vi "SW_Load_parameter_group_3.vi"(0 "Settings file refnum in":T2, 5 "Researcher name in":string, 7 "Settings parameter name":T1, 11 "error in":errorcluster) -> (4 "Settings file refnum out":T2, 6 "Researcher name out":string, 8 "Found?":bool, 10 "Group (section) cluster data out":variant, 15 "error out":errorcluster)   [LabVIEW 2018, in "Tracker.lvlib"]
uses:
  Tracker.lvlib
  <vilib>/Utility/config.llb/Config Data RefNum.ctl
  Controls/CTL_Settings_parameter_group_enum.ctl
  Controls/CTL_Settings_cluster.ctl
  Controls/CTL_Histogram_parameters.ctl
  Controls/CTL_Filter_selector.ctl
  Controls/CTL_Acquisition_speed_selector.ctl
  Controls/CTL_Segmented_plot_parameters.ctl
  Controls/CTL_IO_params_cluster.ctl
  Controls/CTL_Conditions_Array.ctl
  Controls/CTL_Conditions_Cluster.ctl
  Controls/CTL_Condition_type.ctl
  Controls/CTL_Comparison_type.ctl
  Controls/CTL_Validity_check_criteria.ctl
  Controls/CTL_Response_info.ctl
  Controls/CTL_Condition_response_type.ctl
  Controls/CTL_Reponse_port_info.ctl
  Controls/CTL_Calibration_parameters.ctl
  Controls/CTL_Dispenser_calibration_info.ctl
  Controls/CTL_Conditions_All_Presets_Cluster.ctl
  <vilib>/Utility/config.llb/NI_LVConfig.lvlib
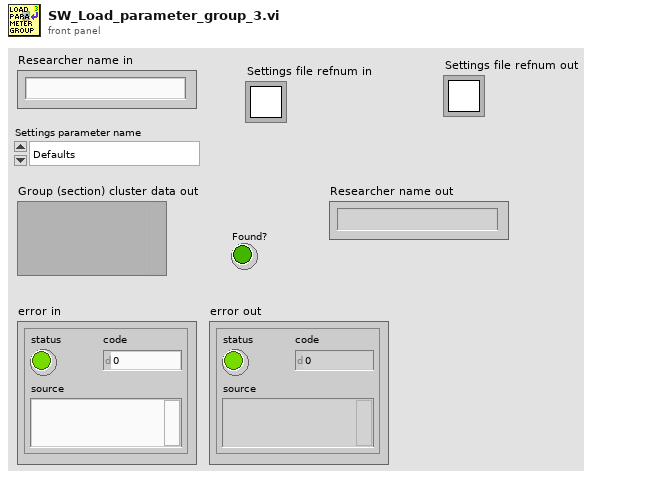
[diagram p1: front panel]
types:
  T1 = typedef "Tracker.lvlib/CTL_Settings_parameter_group_enum.ctl" = enum16{"Defaults", "Recording and saving", "Geometry", "IO parameters", "Conditions presets array (gzip)", "Conditions presets array", "Calibration", "All"}
  T2 = typedef "NI_LVConfig.lvlib/Config Data RefNum.ctl" = refnum<k1>
  T3 = typedef "Tracker.lvlib/CTL_Settings_cluster.ctl" = cluster{"Defaults":cluster{"Default User":dbl, "VISA Resource Name ":string, "Histogram parameters":T4}, "Recording and saving":cluster{"Researcher name":string, "Name prefix":string, "Data post-processing":T5, "Stop at":dbl, "\"Stop at\" enabled":bool, "Default save folder path":path, "Acquisition FPS":T6}, "Geometry":T7, "IO parameters":T8, "Conditions presets array":T9, "Calibration parameters":T17, "Settings loaded OK":bool}
  T4 = typedef "Tracker.lvlib/CTL_Histogram_parameters.ctl" = cluster{"max":dbl, "min":dbl, "# bins":i32, "threshold":dbl, "thr. type":enum16{"higher accepted", "lower accepted"}}
  T5 = typedef "Tracker.lvlib/CTL_Filter_selector.ctl" = cluster{"Filter type":enum16{"None", "Savitzky-Golay"}, "Length":i32, "Order":i32}
  T6 = typedef "Tracker.lvlib/CTL_Acquisition_speed_selector.ctl" = enum16{"Max", "Optimal", "Eco"}
  T7 = typedef "Tracker.lvlib/CTL_Segmented_plot_parameters.ctl" = cluster{"Cage diameter, mm":u16, "Starting angle MIDFIELD":i16, "Starting angle BORDER":i16, "Radius, mm CENTER":u16, "Radius, mm MIDFIELD":u16, "N segments MIDFIELD":u8, "N segments BORDER":u8, "R-gap, mm":sgl, "Bridge swap":bool, "Bridge H. offset":sgl, "Bridge V. offset":sgl, "Twisted neck":bool, "Alt. magn. orientation":bool, "Sensor board size":enum16{"Small", "Large"}}
  T8 = typedef "Tracker.lvlib/CTL_IO_params_cluster.ctl" = cluster{"IO general config.":u16, "IO 1 configuration":u16, "IO 2 configuration":u16, "IO 3 configuration":u16, "IO 4 configuration":u16, "Activate ext. RS-232":u16, "IO inversion config.":u16, "Sync capability":u8}
  T9 = typedef "Tracker.lvlib/CTL_Conditions_Array.ctl" = T10[]
  T10 = typedef "Tracker.lvlib/CTL_Conditions_Cluster.ctl" = cluster{"Enabled":bool, "Name":string, "Specifier(s)":cluster{"Specifier enabled":bool, "Condition type":T11, "Comparison type":T12, "Value":dbl, "Validity criteria(s)":cluster{"V. check enabled":bool, "Criteria":T13, "Validity value":dbl}[]}[], "Response":T14, "Has been set":bool}
  T11 = typedef "Tracker.lvlib/CTL_Condition_type.ctl" = enum16{"Speed", "Zone", "Angle to wall"}
  T12 = typedef "Tracker.lvlib/CTL_Comparison_type.ctl" = enum16{"Less", "Less or Equal", "Equal", "Greater or Equal", "Greater", "Not Equal"}
  T13 = typedef "Tracker.lvlib/CTL_Validity_check_criteria.ctl" = enum16{"Running bout (seconds)", "Running bout (meters)"}
  T14 = typedef "Tracker.lvlib/CTL_Response_info.ctl" = cluster{"Response type":T15, "TTL port":T16, "TTL pulse length, ms":dbl}
  T15 = typedef "Tracker.lvlib/CTL_Condition_response_type.ctl" = enum16{"None", "Air puff", "Liquid reward"}
  T16 = typedef "Tracker.lvlib/CTL_Reponse_port_info.ctl" = enum16{"Port 1", "Port 2", "Port 3", "Port 4"}
  T17 = typedef "Tracker.lvlib/CTL_Calibration_parameters.ctl" = cluster{"Timing calibration sw/hw":dbl, "True FPS":dbl, "True frame time, s":dbl, "Disp. calibration info":T18}
  T18 = typedef "Tracker.lvlib/CTL_Dispenser_calibration_info.ctl" = cluster{"Channel":u8, "Speed, µl per ms":dbl}[]
  T19 = typedef "Tracker.lvlib/CTL_Conditions_All_Presets_Cluster.ctl" = cluster{"[0]":string, "[1]":string, "[2]":string, "[3]":string, "[4]":string, "[5]":string, "[6]":string, "[7]":string, "[8]":string}
  T20 = cluster{"Default User":dbl, "VISA Resource Name ":string, "Histogram parameters":T4}
  T21 = cluster{"Researcher name":string, "Name prefix":string, "Data post-processing":T5, "Stop at":dbl, "\"Stop at\" enabled":bool, "Default save folder path":path, "Acquisition FPS":T6}
  T22 = cluster{"Conditions presets array[0]":T10, "Conditions presets array[1]":T10, "Conditions presets array[2]":T10, "Conditions presets array[3]":T10, "Conditions presets array[4]":T10, "Conditions presets array[5]":T10, "Conditions presets array[6]":T10, "Conditions presets array[7]":T10, "Conditions presets array[8]":T10}
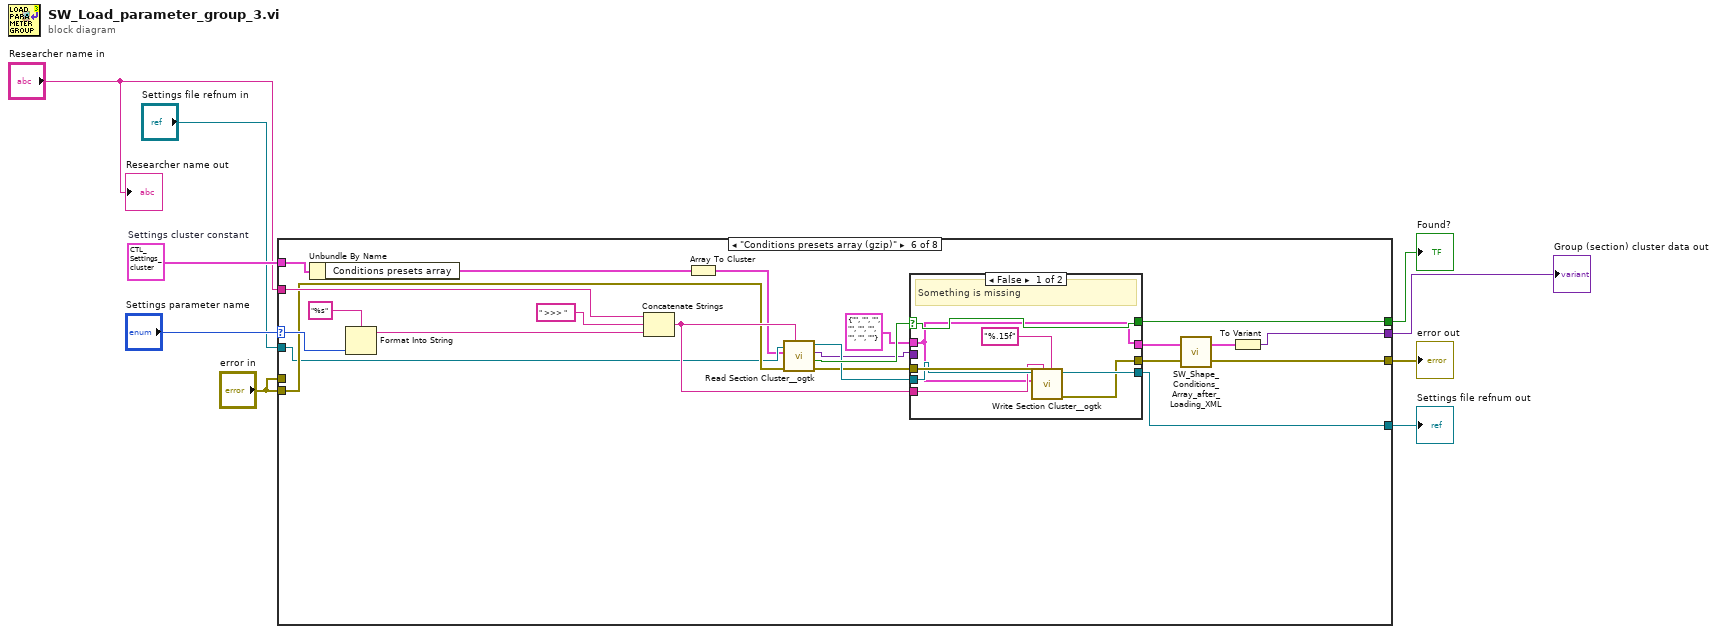
[diagram p0: block diagram]
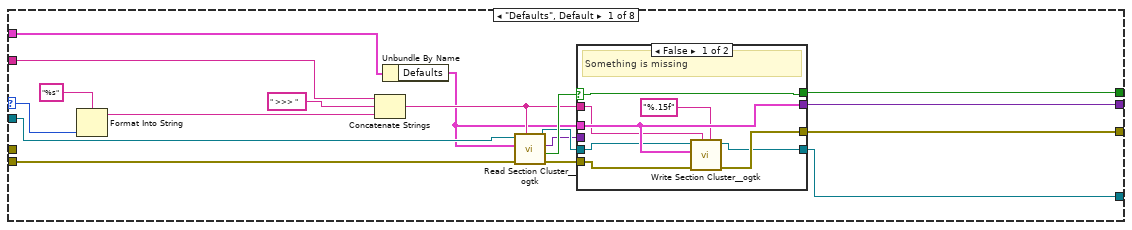
[diagram p2: hidden frame]
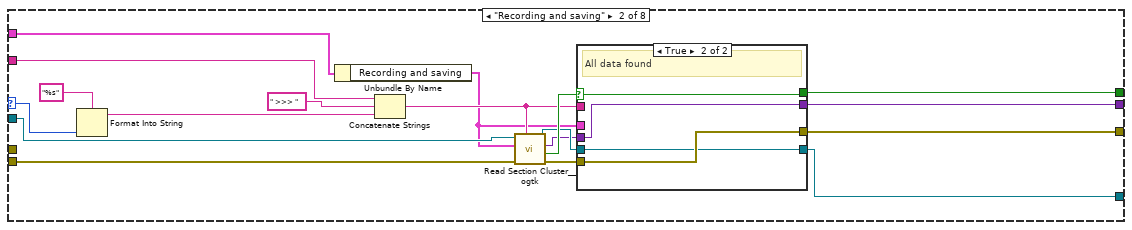
[diagram p4: hidden frame]
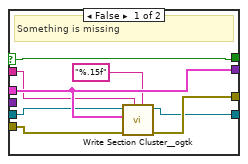
[diagram p5: hidden frame]
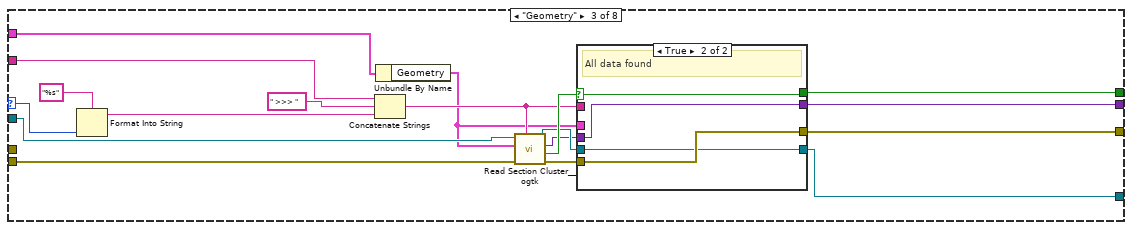
[diagram p6: hidden frame]
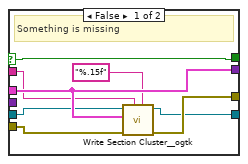
[diagram p7: hidden frame]
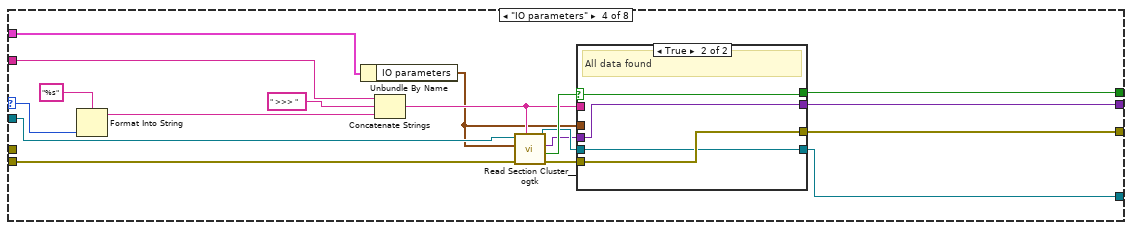
[diagram p8: hidden frame]
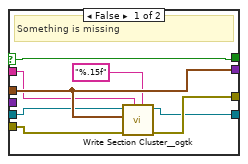
[diagram p9: hidden frame]
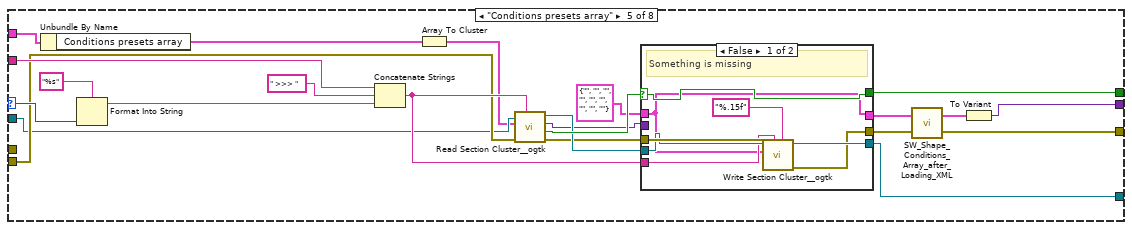
[diagram p10: hidden frame]
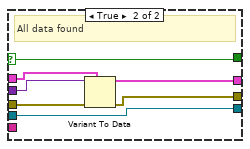
[diagram p11: hidden frame]
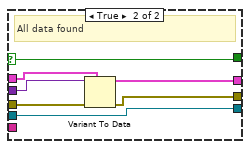
[diagram p12: hidden frame]
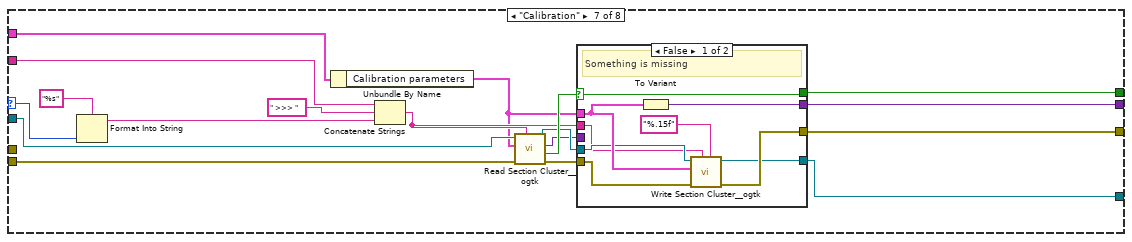
[diagram p13: hidden frame]
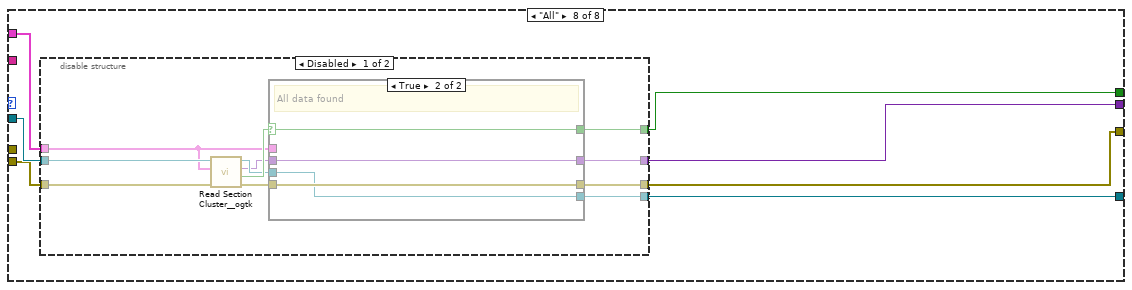
[diagram p15: hidden frame]
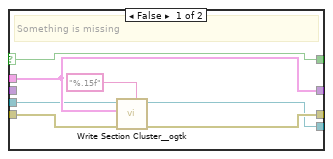
[diagram p16: hidden frame]
diagram:
  w5 = T3 {"Defaults"={"Default User"=0.0, "VISA Resource Name "="", "Histogram parameters"={"max"=300.0, "min"=0.0, "# bins"=10, "threshold"=8.0, "thr. type"=enum."higher accepted"}}, "Recording and saving"={"Researcher name"="Researcher", "Name prefix"="Track", "Data post-processing"={"Filter type"=enum."Savitzky-Golay", "Length"=31, "Order"=3}, "Stop at"=0.0, "\"Stop at\" enabled"=FALSE, "Default save folder path"=path "", "Acquisition FPS"=enum."Max"}, "Geometry"={"Cage diameter, mm"=180, "Starting angle MIDFIELD"=0, "Starting angle BORDER"=0, "Radius, mm CENTER"=30, "Radius, mm MIDFIELD"=75, "N segments MIDFIELD"=2, "N segments BORDER"=4, "R-gap, mm"=0.0, "Bridge swap"=FALSE, "Bridge H. offset"=0.0, "Bridge V. offset"=0.0, "Twisted neck"=FALSE, "Alt. magn. orientation"=FALSE, "Sensor board size"=enum."Small"}, "IO parameters"={"IO general config."=12, "IO 1 configuration"=1, "IO 2 configuration"=1, "IO 3 configuration"=0, "IO 4 configuration"=0, "Activate ext. RS-232"=0, "IO inversion config."=0, "Sync capability"=1}, "Conditions presets array"=[{"Enabled"=FALSE, "Name"="", "Specifier(s)"=[], "Response"={"Response type"=enum."Air puff", "TTL port"=enum."Port 1", "TTL pulse length, ms"=0.0}, "Has been set"=FALSE}, {"Enabled"=FALSE, "Name"="", "Specifier(s)"=[], "Response"={"Response type"=enum."Air puff", "TTL port"=enum."Port 1", "TTL pulse length, ms"=0.0}, "Has been set"=FALSE}, {"Enabled"=FALSE, "Name"="", "Specifier(s)"=[], "Response"={"Response type"=enum."Air puff", "TTL port"=enum."Port 1", "TTL pulse length, ms"=0.0}, "Has been set"=FALSE}, {"Enabled"=FALSE, "Name"="", "Specifier(s)"=[], "Response"={"Response type"=enum."Air puff", "TTL port"=enum."Port 1", "TTL pulse length, ms"=0.0}, "Has been set"=FALSE}, {"Enabled"=FALSE, "Name"="", "Specifier(s)"=[], "Response"={"Response type"=enum."Air puff", "TTL port"=enum."Port 1", "TTL pulse length, ms"=0.0}, "Has been set"=FALSE}, {"Enabled"=FALSE, "Name"="", "Specifier(s)"=[], "Response"={"Response type"=enum."Air puff", "TTL port"=enum."Port 1", "TTL pulse length, ms"=0.0}, "Has been set"=FALSE}, {"Enabled"=FALSE, "Name"="", "Specifier(s)"=[], "Response"={"Response type"=enum."Air puff", "TTL port"=enum."Port 1", "TTL pulse length, ms"=0.0}, "Has been set"=FALSE}, {"Enabled"=FALSE, "Name"="", "Specifier(s)"=[], "Response"={"Response type"=enum."Air puff", "TTL port"=enum."Port 1", "TTL pulse length, ms"=0.0}, "Has been set"=FALSE}, {"Enabled"=FALSE, "Name"="", "Specifier(s)"=[], "Response"={"Response type"=enum."Air puff", "TTL port"=enum."Port 1", "TTL pulse length, ms"=0.0}, "Has been set"=FALSE}, {"Enabled"=FALSE, "Name"="", "Specifier(s)"=[], "Response"={"Response type"=enum."Air puff", "TTL port"=enum."Port 1", "TTL pulse length, ms"=0.0}, "Has been set"=FALSE}, {"Enabled"=FALSE, "Name"="", "Specifier(s)"=[], "Response"={"Response type"=enum."Air puff", "TTL port"=enum."Port 1", "TTL pulse length, ms"=0.0}, "Has been set"=FALSE}, {"Enabled"=FALSE, "Name"="", "Specifier(s)"=[], "Response"={"Response type"=enum."Air puff", "TTL port"=enum."Port 1", "TTL pulse length, ms"=0.0}, "Has been set"=FALSE}, {"Enabled"=FALSE, "Name"="", "Specifier(s)"=[], "Response"={"Response type"=enum."Air puff", "TTL port"=enum."Port 1", "TTL pulse length, ms"=0.0}, "Has been set"=FALSE}, {"Enabled"=FALSE, "Name"="", "Specifier(s)"=[], "Response"={"Response type"=enum."Air puff", "TTL port"=enum."Port 1", "TTL pulse length, ms"=0.0}, "Has been set"=FALSE}], "Calibration parameters"={"Timing calibration sw/hw"=1.0, "True FPS"=80.0, "True frame time, s"=80.0, "Disp. calibration info"=[{"Channel"=1, "Speed, µl per ms"=1.0}, {"Channel"=2, "Speed, µl per ms"=1.0}, {"Channel"=3, "Speed, µl per ms"=1.0}, {"Channel"=4, "Speed, µl per ms"=1.0}]}, "Settings loaded OK"=FALSE}  # Settings cluster constant
  n1 = case shown="\"Conditions presets array (gzip)\"" "Settings parameter name" {
    selector: "Settings parameter name" -> [w16 w46 w76 w106 w149 w187 w212 _]
    tunnel: [w23 w53 w83 w113 w145 w183 w219 w243] -> w9
    tunnel: [w22 w52 w82 w112 w131 w169 w218 w242] -> w8
    tunnel: [w20 w50 w80 w110 w135 w173 w216 w241] -> w7
    tunnel: "Researcher name in" -> [w15 w45 w75 w105 w148 w186 w211 _]
    tunnel: "Settings file refnum in" -> [w14 w44 w74 w104 w137 w175 w210 w240]
    tunnel: "error in" -> [w13 w43 w73 w103 w138 w176 w209 w239]
    tunnel: w5 -> [w12 w42 w72 w102 w147 w185 w208 w237]
    tunnel: [w10 w40 w70 w100 w146 w184 w206 w238] -> w4
    tunnel: "error in" -> [_ _ _ _ _ _ _ _]
    frame "Defaults", Default {
      n2 = Format Into String(format string="%s", w16) -> (resulting string=w17:string)  [unwired: 2 in, 1 out]
      n3 = Concatenate Strings(w15, " >>> " ("string"), w17) -> (w19:string)
      n4 = Unbundle By Name(w12) -> ("Defaults"=w11:T20)
      n5 = call <userlib>:"Read Section Cluster__ogtk.vi"("section (optional)"=w19, "error in (no error)"=w13, "Section Formatted Cluster Type"=w11, "refnum"=w14) -> ("error out"=w24:errorcluster, "all found?"=w26:bool, "Section Formatted Cluster"=w21:variant, "dup refnum"=w25:T2)  [unwired: 3 in, 1 out]
      n6 = case shown="False" w26 {
        selector: w26 -> [w28 w36]
        tunnel: w25 -> [w32 w38]
        tunnel: w24 -> [w35 w39]
        tunnel: [w34 w39] -> w22
        tunnel: [w31 w38] -> w23
        tunnel: w21 -> [_ w37]
        tunnel: [w33 w37] -> w20
        tunnel: w11 -> [w33 _]
        tunnel: w19 -> [w30 _]
        tunnel: [w28 w36] -> w10
        frame False {
          # "Something is missing"
          n7 = call <userlib>:"Write Section Cluster__ogtk.vi"("float number format (optional)"="%.15f", "section (optional)"=w30, "error in (no error)"=w35, "Section Formatted Cluster"=w33, "refnum"=w32) -> ("error out"=w34:errorcluster, "dup refnum"=w31:T2)  [unwired: 5 in]
        }
        frame True {
          # "All data found"
        }
      }
    }
    frame "Recording and saving" {
      n8 = Format Into String(format string="%s", w46) -> (resulting string=w47:string)  [unwired: 2 in, 1 out]
      n9 = Unbundle By Name(w42) -> ("Recording and saving"=w41:T21)
      n10 = Concatenate Strings(w45, " >>> " ("string"), w47) -> (w49:string)
      n11 = call <userlib>:"Read Section Cluster__ogtk.vi"("section (optional)"=w49, "error in (no error)"=w43, "Section Formatted Cluster Type"=w41, "refnum"=w44) -> ("error out"=w54:errorcluster, "all found?"=w56:bool, "Section Formatted Cluster"=w51:variant, "dup refnum"=w55:T2)  [unwired: 3 in, 1 out]
      n12 = case shown="True" w56 {
        selector: w56 -> [w58 w66]
        tunnel: w55 -> [w62 w68]
        tunnel: w54 -> [w65 w69]
        tunnel: [w64 w69] -> w52
        tunnel: [w61 w68] -> w53
        tunnel: w51 -> [_ w67]
        tunnel: [w63 w67] -> w50
        tunnel: w41 -> [w63 _]
        tunnel: w49 -> [w60 _]
        tunnel: [w58 w66] -> w40
        frame False {
          # "Something is missing"
          n13 = call <userlib>:"Write Section Cluster__ogtk.vi"("float number format (optional)"="%.15f", "section (optional)"=w60, "error in (no error)"=w65, "Section Formatted Cluster"=w63, "refnum"=w62) -> ("error out"=w64:errorcluster, "dup refnum"=w61:T2)  [unwired: 5 in]
        }
        frame True {
          # "All data found"
        }
      }
    }
    frame "Geometry" {
      n14 = Format Into String(format string="%s", w76) -> (resulting string=w77:string)  [unwired: 2 in, 1 out]
      n15 = Concatenate Strings(w75, " >>> " ("string"), w77) -> (w79:string)
      n16 = Unbundle By Name(w72) -> ("Geometry"=w71:T7)
      n17 = call <userlib>:"Read Section Cluster__ogtk.vi"("section (optional)"=w79, "error in (no error)"=w73, "Section Formatted Cluster Type"=w71, "refnum"=w74) -> ("error out"=w84:errorcluster, "all found?"=w86:bool, "Section Formatted Cluster"=w81:variant, "dup refnum"=w85:T2)  [unwired: 3 in, 1 out]
      n18 = case shown="True" w86 {
        selector: w86 -> [w88 w96]
        tunnel: w85 -> [w92 w98]
        tunnel: w84 -> [w95 w99]
        tunnel: [w94 w99] -> w82
        tunnel: [w91 w98] -> w83
        tunnel: w81 -> [_ w97]
        tunnel: [w93 w97] -> w80
        tunnel: w71 -> [w93 _]
        tunnel: w79 -> [w90 _]
        tunnel: [w88 w96] -> w70
        frame False {
          # "Something is missing"
          n19 = call <userlib>:"Write Section Cluster__ogtk.vi"("float number format (optional)"="%.15f", "section (optional)"=w90, "error in (no error)"=w95, "Section Formatted Cluster"=w93, "refnum"=w92) -> ("error out"=w94:errorcluster, "dup refnum"=w91:T2)  [unwired: 5 in]
        }
        frame True {
          # "All data found"
        }
      }
    }
    frame "IO parameters" {
      n20 = Format Into String(format string="%s", w106) -> (resulting string=w107:string)  [unwired: 2 in, 1 out]
      n21 = Unbundle By Name(w102) -> ("IO parameters"=w101:T8)
      n22 = Concatenate Strings(w105, " >>> " ("string"), w107) -> (w109:string)
      n23 = call <userlib>:"Read Section Cluster__ogtk.vi"("section (optional)"=w109, "error in (no error)"=w103, "Section Formatted Cluster Type"=w101, "refnum"=w104) -> ("error out"=w114:errorcluster, "all found?"=w116:bool, "Section Formatted Cluster"=w111:variant, "dup refnum"=w115:T2)  [unwired: 3 in, 1 out]
      n24 = case shown="True" w116 {
        selector: w116 -> [w118 w126]
        tunnel: w115 -> [w122 w128]
        tunnel: w114 -> [w125 w129]
        tunnel: [w124 w129] -> w112
        tunnel: [w121 w128] -> w113
        tunnel: w111 -> [_ w127]
        tunnel: [w123 w127] -> w110
        tunnel: w101 -> [w123 _]
        tunnel: w109 -> [w120 _]
        tunnel: [w118 w126] -> w100
        frame False {
          # "Something is missing"
          n25 = call <userlib>:"Write Section Cluster__ogtk.vi"("float number format (optional)"="%.15f", "section (optional)"=w120, "error in (no error)"=w125, "Section Formatted Cluster"=w123, "refnum"=w122) -> ("error out"=w124:errorcluster, "dup refnum"=w121:T2)  [unwired: 5 in]
        }
        frame True {
          # "All data found"
        }
      }
    }
    frame "Conditions presets array" {
      n26 = Unbundle By Name(w147) -> ("Conditions presets array"=w143:T9)
      n27 = Format Into String(format string="%s", w149) -> (resulting string=w150:string)  [unwired: 2 in, 1 out]
      n28 = Concatenate Strings(w148, " >>> " ("string"), w150) -> (w144:string)
      n29 = Array To Cluster(array=w143) -> (cluster=w130:T22)
      n30 = call <userlib>:"Read Section Cluster__ogtk.vi"("section (optional)"=w144, "error in (no error)"=w138, "Section Formatted Cluster Type"=w130, "refnum"=w137) -> ("error out"=w140:errorcluster, "all found?"=w142:bool, "Section Formatted Cluster"=w139:variant, "dup refnum"=w141:T2)  [unwired: 3 in, 1 out]
      n31 = case shown="False" w142 {
        selector: w142 -> [w155 w166]
        tunnel: w141 -> [w159 w167]
        tunnel: w140 -> [w160 w165]
        tunnel: [w154 w161] -> w134
        tunnel: [w158 w167] -> w145
        tunnel: w139 -> [_ w164]
        tunnel: w144 -> [w157 _]
        tunnel: [w155 w166] -> w146
        tunnel: T19 {"[0]"="", "[1]"="", "[2]"="", "[3]"="", "[4]"="", "[5]"="", "[6]"="", "[7]"="", "[8]"=""} ("Condition presets prepared for saving out") -> [w153 w163]
        tunnel: [w153 w162] -> w133
        frame False {
          # "Something is missing"
          n32 = call <userlib>:"Write Section Cluster__ogtk.vi"("float number format (optional)"="%.15f", "section (optional)"=w157, "error in (no error)"=w160, "Section Formatted Cluster"=w153, "refnum"=w159) -> ("error out"=w154:errorcluster, "dup refnum"=w158:T2)  [unwired: 5 in]
        }
        frame True {
          # "All data found"
          n33 = Variant To Data(error in=w165, type=w163, Variant=w164) -> (data=w162:T19, error out=w161:errorcluster)
        }
      }
      n34 = call "SW_Shape_Conditions_Array_after_Loading_XML.vi"("error in (no error)"=w134, "Condition presets loaded in"=w133) -> ("error out"=w131:errorcluster, "Conditions presets array out"=w132:T9)
      n35 = To Variant(anything=w132) -> (Variant=w135:variant)
    }
    frame "Conditions presets array (gzip)" {
      n36 = Unbundle By Name(w185) -> ("Conditions presets array"=w181:T9)
      n37 = Format Into String(format string="%s", w187) -> (resulting string=w188:string)  [unwired: 2 in, 1 out]
      n38 = Concatenate Strings(w186, " >>> " ("string"), w188) -> (w182:string)
      n39 = Array To Cluster(array=w181) -> (cluster=w168:T22)
      n40 = call <userlib>:"Read Section Cluster__ogtk.vi"("section (optional)"=w182, "error in (no error)"=w176, "Section Formatted Cluster Type"=w168, "refnum"=w175) -> ("error out"=w178:errorcluster, "all found?"=w180:bool, "Section Formatted Cluster"=w177:variant, "dup refnum"=w179:T2)  [unwired: 3 in, 1 out]
      n41 = case shown="False" w180 {
        selector: w180 -> [w193 w204]
        tunnel: w179 -> [w197 w205]
        tunnel: w178 -> [w198 w203]
        tunnel: [w192 w199] -> w172
        tunnel: [w196 w205] -> w183
        tunnel: w177 -> [_ w202]
        tunnel: w182 -> [w195 _]
        tunnel: [w193 w204] -> w184
        tunnel: T19 {"[0]"="", "[1]"="", "[2]"="", "[3]"="", "[4]"="", "[5]"="", "[6]"="", "[7]"="", "[8]"=""} ("Condition presets prepared for saving out") -> [w191 w201]
        tunnel: [w191 w200] -> w171
        frame False {
          # "Something is missing"
          n42 = call <userlib>:"Write Section Cluster__ogtk.vi"("float number format (optional)"="%.15f", "section (optional)"=w195, "error in (no error)"=w198, "Section Formatted Cluster"=w191, "refnum"=w197) -> ("error out"=w192:errorcluster, "dup refnum"=w196:T2)  [unwired: 5 in]
        }
        frame True {
          # "All data found"
          n43 = Variant To Data(error in=w203, type=w201, Variant=w202) -> (data=w200:T19, error out=w199:errorcluster)
        }
      }
      n44 = call "SW_Shape_Conditions_Array_after_Loading_XML.vi"("error in (no error)"=w172, "Condition presets loaded in"=w171) -> ("error out"=w169:errorcluster, "Conditions presets array out"=w170:T9)
      n45 = To Variant(anything=w170) -> (Variant=w173:variant)
    }
    frame "Calibration" {
      n46 = Format Into String(format string="%s", w212) -> (resulting string=w213:string)  [unwired: 2 in, 1 out]
      n47 = Unbundle By Name(w208) -> ("Calibration parameters"=w207:T17)
      n48 = Concatenate Strings(w211, " >>> " ("string"), w213) -> (w215:string)
      n49 = call <userlib>:"Read Section Cluster__ogtk.vi"("section (optional)"=w215, "error in (no error)"=w209, "Section Formatted Cluster Type"=w207, "refnum"=w210) -> ("error out"=w220:errorcluster, "all found?"=w222:bool, "Section Formatted Cluster"=w217:variant, "dup refnum"=w221:T2)  [unwired: 3 in, 1 out]
      n50 = case shown="False" w222 {
        selector: w222 -> [w225 w233]
        tunnel: w221 -> [w229 w235]
        tunnel: w220 -> [w232 w236]
        tunnel: [w231 w236] -> w218
        tunnel: [w228 w235] -> w219
        tunnel: w217 -> [_ w234]
        tunnel: [w224 w234] -> w216
        tunnel: w207 -> [w230 _]
        tunnel: w215 -> [w227 _]
        tunnel: [w225 w233] -> w206
        frame False {
          # "Something is missing"
          n51 = To Variant(anything=w230) -> (Variant=w224:variant)
          n52 = call <userlib>:"Write Section Cluster__ogtk.vi"("float number format (optional)"="%.15f", "section (optional)"=w227, "error in (no error)"=w232, "Section Formatted Cluster"=w230, "refnum"=w229) -> ("error out"=w231:errorcluster, "dup refnum"=w228:T2)  [unwired: 5 in]
        }
        frame True {
          # "All data found"
        }
      }
    }
    frame "All" {
      n53 = disable-structure shown="Disabled" {
        disable-tunnel: [w251 _] -> w243
        disable-tunnel: [w250 _] -> w242
        disable-tunnel: [w248 _] -> w241
        disable-tunnel: w240 -> [w247 _]
        disable-tunnel: w239 -> [w246 _]
        disable-tunnel: [w245 _] -> w238
        disable-tunnel: w237 -> [w244 _]
        frame Disabled {
          n54 = call <userlib>:"Read Section Cluster__ogtk.vi"("error in (no error)"=w246, "Section Formatted Cluster Type"=w244, "refnum"=w247) -> ("error out"=w252:errorcluster, "all found?"=w254:bool, "Section Formatted Cluster"=w249:variant, "dup refnum"=w253:T2)  [unwired: 4 in, 1 out]
          n55 = case shown="True" w254 {
            selector: w254 -> [w255 w262]
            tunnel: w253 -> [w258 w264]
            tunnel: w252 -> [w261 w265]
            tunnel: [w260 w265] -> w250
            tunnel: [w257 w264] -> w251
            tunnel: w249 -> [_ w263]
            tunnel: [w259 w263] -> w248
            tunnel: w244 -> [w259 _]
            tunnel: [w255 w262] -> w245
            frame False {
              # "Something is missing"
              n56 = call <userlib>:"Write Section Cluster__ogtk.vi"("float number format (optional)"="%.15f", "error in (no error)"=w261, "Section Formatted Cluster"=w259, "refnum"=w258) -> ("error out"=w260:errorcluster, "dup refnum"=w257:T2)  [unwired: 6 in]
            }
            frame True {
              # "All data found"
            }
          }
        }
        frame Enabled {
        }
      }
    }
  }
  "error out" <- w8
  "Settings file refnum out" <- w9
  "Group (section) cluster data out" <- w7
  "Found?" <- w4
  "Researcher name out" <- "Researcher name in"
